vi "XLP80_HH_Main.vi"(8 "err in":errorcluster) -> (0 "err out":errorcluster)   [LabVIEW 2021]
uses:
  XLP80_Globals/Globals_Settings_XLP80.vi
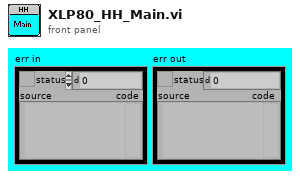
[diagram p1: front panel]
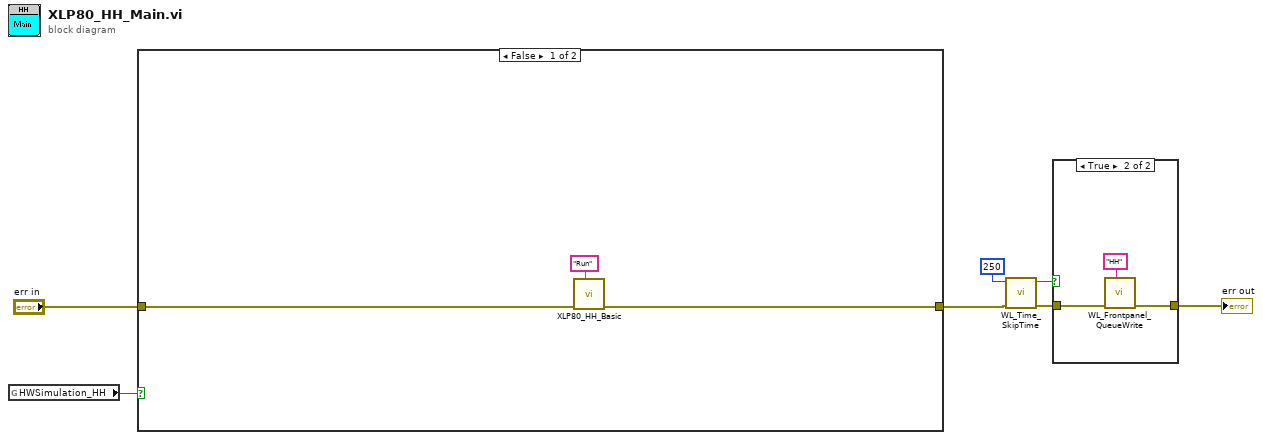
[diagram p0: block diagram]
diagram:
  n1 = global read "Globals_Settings_XLP80.vi" "HWSimulation_HH"() -> (w1:bool)
  n2 = case shown="False" w1 {
    tunnel: "err in" -> [w10 w11]
    tunnel: [w9 w11] -> w2
    frame False {
      n3 = call "XLP80_HH_Basic.vi"("Function"="Run", "err in"=w10) -> ("err out"=w9:errorcluster)  [unwired: 9 in]
    }
    frame True {
    }
  }
  n4 = call "WL_Time_SkipTime.vi"("err in"=w2, "SkipTime[ms]"=u32 250) -> ("err out"=w6:errorcluster, "Run"=w5:bool)  [unwired: 8 in]
  n5 = case shown="True" w5 {
    tunnel: [w12 w15] -> w3
    tunnel: w6 -> [w12 w14]
    frame False {
    }
    frame True {
      n6 = call "WL_Frontpanel_QueueWrite.vi"("Command (error only)"="HH", "err in"=w14) -> ("err out"=w15:errorcluster)  [unwired: 9 in]
    }
  }
  "err out" <- w3
